vi "Intake_set.vi"   [LabVIEW 2020]
uses:
  Globals/Intake_Globals.vi
  Intake_control_states.ctl
types:
  T1 = typedef "Intake_control_states.ctl" = enum16{"No_Op", "Intake", "Manual", "Outtake"}
  T2 = typedef "Intake_cluster.ctl" = cluster{"control_states":T1, "%Vbus":dbl, "Trigger?":bool, "Manual_Extend?":bool, "Auto_Notifier":refnum<notifier>, "Step":dbl, "Parameter 1":dbl, "Parameter 2":dbl, "Parameter 3":dbl}
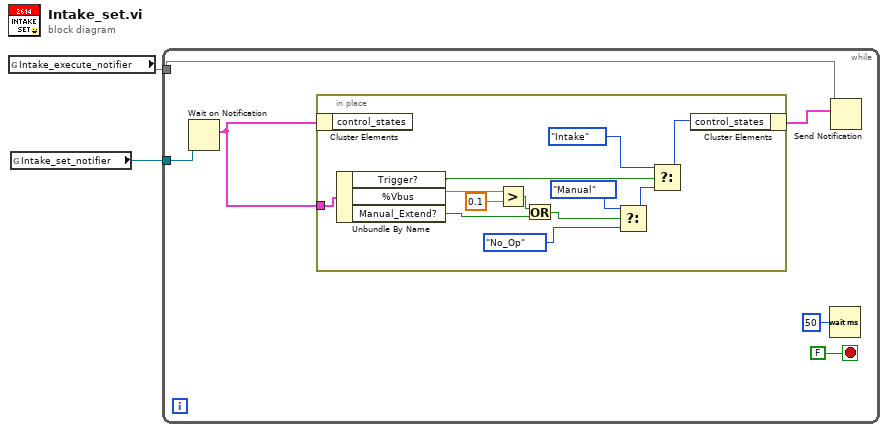
[diagram p0: block diagram]
diagram:
  n1 = global read "Intake_Globals.vi" "Intake_execute_notifier"() -> (w2)
  n2 = global read "Intake_Globals.vi" "Intake_set_notifier"() -> (w1:refnum<notifier>)
  n3 = while {
    tunnel: w1 -> [w8]
    tunnel: w2 -> [w5]
    stop <- FALSE stop-if-true
    n4 = Wait on Notification(notifier=w8) -> (notification=w3:T2)  [unwired: 3 in, 3 out]
    n5 = in-place {
      in-place-border: w3 -> [w18]
      n6 = in-place-cluster #1(w3) -> ()  [unwired: 1 out]
      n7 = Unbundle By Name(w18) -> ("Trigger?"=w17:bool, "%Vbus"=w15:dbl, "Manual_Extend?"=w12:bool)
      n8 = Greater?(x=w15, y=0.1) -> (0:w13:bool)
      n9 = Or(x=w13, y=w12) -> (x .or. y?=w11:bool)
      n10 = Select(t=Intake_control_states."Manual", s=w11, f=Intake_control_states."No_Op" ("control_states")) -> (s? t:f=w9:T1)
      n11 = Select(t=Intake_control_states."Intake" ("control_states"), s=w17, f=w9) -> (s? t:f=w19:T1)
      n12 = in-place-cluster #1("control_states"=w19) -> (w4:T2)
    }
    n13 = Wait (ms)(milliseconds to wait=u32 50) -> ()  [unwired: 1 out]
    n14 = Send Notification(notification=w4, notifier=w5) -> ()  [unwired: 1 in, 2 out]
  }
